vi "Test Resize ARGB.vi"(8 "error in (no error)":errorcluster, 11 "Test Case In":refnum<class "01_Image.lvclass">) -> (0 "error out":errorcluster, 3 "Test Case Out":refnum<class "01_Image.lvclass">)   [LabVIEW 2020, in "test.lvlib" / "01_Image.lvclass"]
uses:
  01_Image.lvclass
  C:/Program Files (x86)/National Instruments/LabVIEW 2026/vi.lib/Astemes/LUnit/Test Case.lvclass
  common/Image Size (Integer).ctl
  image/Interpolation Mode.ctl
  <vilib>/Astemes/LUnit/Test Case.lvclass/Test Case.ctl
  image/New Image (ARGB Preallocated).vi
  image/Resize (ARGB).vi
  4993e8ee-a06a-463a-9684-69129f64d5ce.vi
  image/Copy Array to Image.vi
  image/Copy Array to Image (ARGB).vi
  image/New Image (ARGB Preallocated).vi/3321fa97-f432-4e1e-8db9-a0df79aed21b.vi
  image/ARGB Colour to U32 Pixel Value.vi
  image/Resize (ARGB).vi/c2d955e4-7b08-44cd-801f-dcd0ae61a3f9.vi
  <vilib>/Astemes/LUnit/Core/LUnit Test Case/Private/Append Pass Result.vi
  <vilib>/Astemes/LUnit/Core/LUnit Test Case/Private/Append Fail Result.vi
  4993e8ee-a06a-463a-9684-69129f64d5ce.vi/9c5d11cd-9439-4240-a1ee-d9baace9c924.vi
  <vilib>/Astemes/LUnit/Core/LUnit Test Case/Private/Run In UI.vi
  <vilib>/Utility/error.llb/Clear Errors.vi
  <vilib>/Utility/error.llb/Error Cluster From Error Code.vi
  <vilib>/picture/pixmap.llb/Flatten Pixmap.vi
  image/image.lvlib
  common/common.lvlib
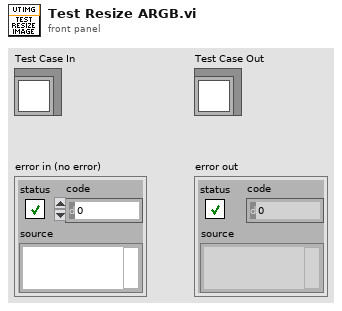
[diagram p1: front panel]
types:
  T1 = typedef "image.lvlib/Interpolation Mode.ctl" = enum8{"NEAREST", "LINEAR", "CUBIC", "AREA", "LANCZOS", "LINEAR_EXACT", "NEAREST_EXACT", "MAX"}
  T2 = typedef "common.lvlib/Image Size (Integer).ctl" = cluster{"Width":u16, "Height":u16}
  T3 = typedef "image.lvlib/ARGB Image.ctl" = refnum<data-value>
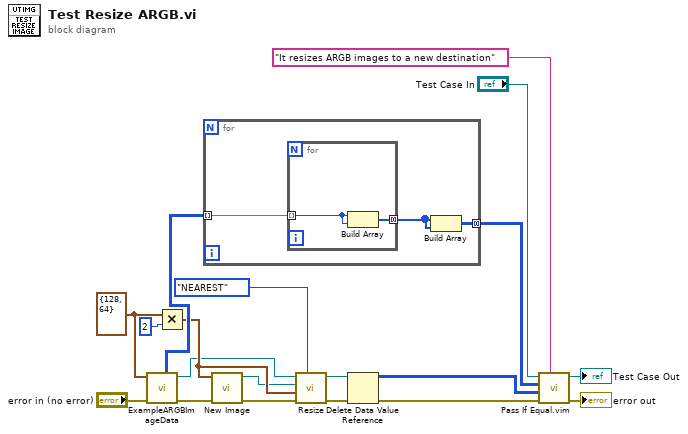
[diagram p0: block diagram]
diagram:
  w11 = T2 {"Width"=128, "Height"=64} ("Preallocated Image Size (Default - 0,0)")
  n1 = call "ExampleARGBImageData.vi"("error in (no error)"="error in (no error)", "Image Size"=w11) -> ("error out"=w5:errorcluster, "Data Value Reference out"=w1:T3, "ARGB Array Data"=w6:u32[][])  [unwired: 6 in, 1 out]
  n2 = Multiply(x=w11, y=u16 2) -> (x*y=w4:T2)
  n3 = for {
    tunnel: w6 -> [w22] mode=indexing
    tunnel: [w20] -> w12 mode=concatenating
    n4 = for {
      tunnel: w22 -> [w24] mode=indexing
      tunnel: [w23] -> w21 mode=concatenating
      n5 = Build Array(w24, w24) -> (w23:u32[])
    }
    n6 = Build Array(w21, w21) -> (w20:u32[][])
  }
  n7 = call-poly "New Image.vi"("error in (no error)"=w5, "Preallocated Image Size (Default: 0,0)"=w4) -> ("error out"=w9:errorcluster, "ARGB Image"=w3:T3)  [unwired: 8 in]
  n8 = call-poly "Resize.vi"("Interpolation Mode (Default: CUBIC)"=Interpolation_Mode."NEAREST" ("OpenCV Interpolation Flag"), "error in (no error)"=w9, "New Image Size"=w4, "ARGB Destination Image in"=w3, "ARGB Source Image in"=w1) -> ("error out"=w2:errorcluster, "ARGB  Destination Image"=w14:T3)  [unwired: 5 in]
  n9 = Delete Data Value Reference(data value reference=w14, error in=w2) -> (data value=w8:u32[][], error out=w16:errorcluster)
  n10 = call "Pass If Equal.vim"("Description"="It resizes ARGB images to a new destination", "error in (no error)"=w16, "Actual"=w8, "Expected"=w12, "LUnit Test Case In"="Test Case In") -> ("error out"=→"error out":errorcluster, "LUnit Test Case Out"=→"Test Case Out":refnum<class "01_Image.lvclass">)  [unwired: 5 in]
